vi "TeachHSLColor.vi"(7 "error in (no error)":errorcluster, 9 "ROI Descriptor":T2 {"Contours"."Type" items=["No Selection", "Point", "Line", "Rectangle", "Oval", "Polygon", "Freehand Region", "Annulus", "Unused2", "Unused3", "Broken Line", "Freehand Line", "Rotated Rectangle"]}, 10 "Image in":T1) -> (0 "error out":errorcluster, 1 "SatLimits":cluster{"Lower value":u8, "Upper value":u8}, 3 "HueLimits":cluster{"Lower value":u8, "Upper value":u8})   [LabVIEW 2015]
uses:
  <vilib>/vision/Image Controls.llb/IMAQ Image.ctl
  <vilib>/vision/NI_Vision_Development_Module.lvlib
panel:
  out "Sat":u32[](graph)
  out "Hue":u32[](graph)
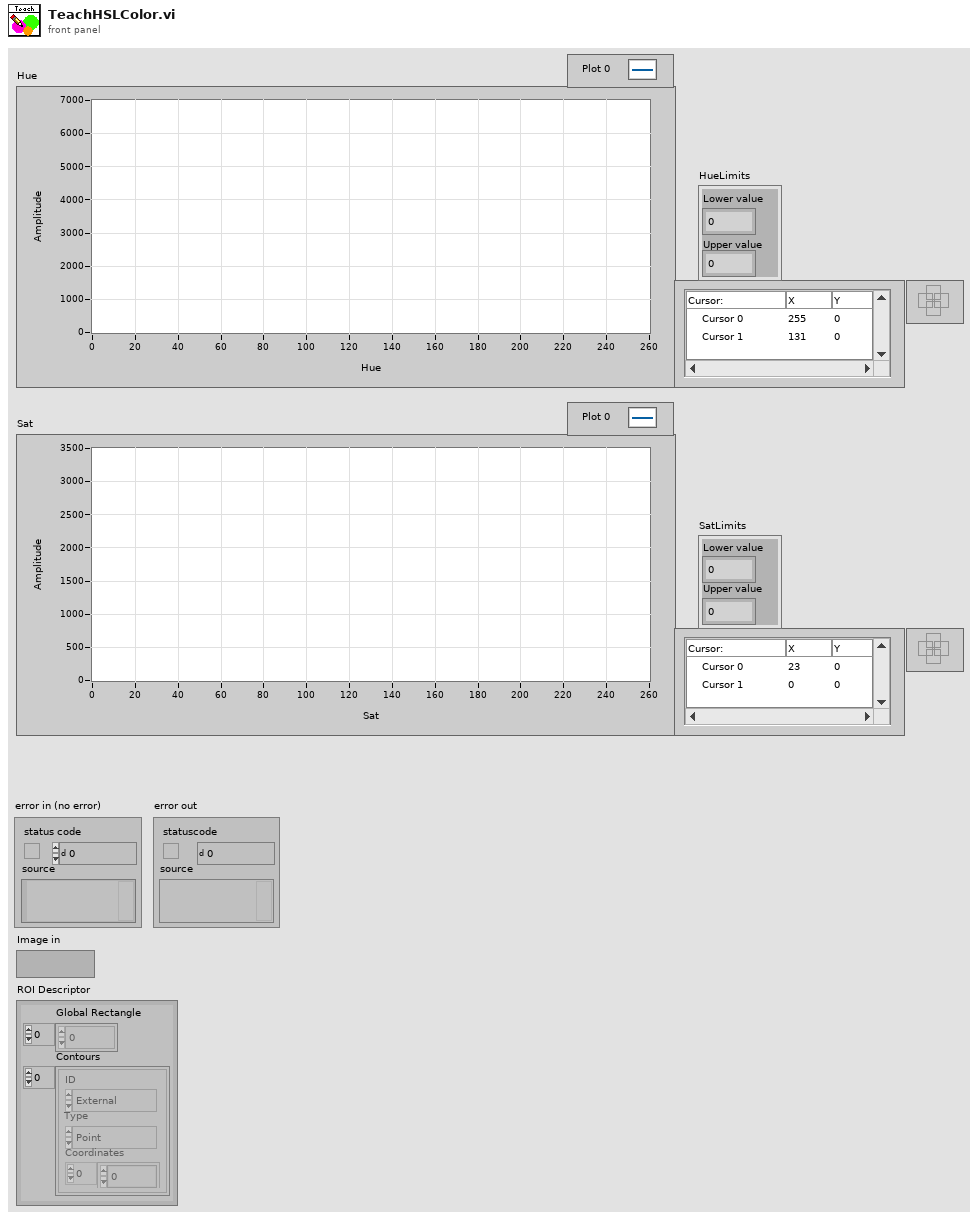
[diagram p1: front panel]
types:
  T1 = typedef "IMAQ Image.ctl" = refnum<image>
  T2 = typedef "ROI Descriptor" = cluster{"Global Rectangle":i32[], "Contours":cluster{"ID":enum32{"External", "Internal"}, "Type":u32, "Coordinates":i32[]}[]}
  T3 = typedef "Image Type" = u32
  T4 = cluster{"histogram":u32[], "Minimal Value":sgl, "Maximal Value":sgl, "Starting Value":sgl, "Interval Width":sgl, "Mean Value":sgl, "Standard  Variation":sgl, "Area (pixels)":i32}
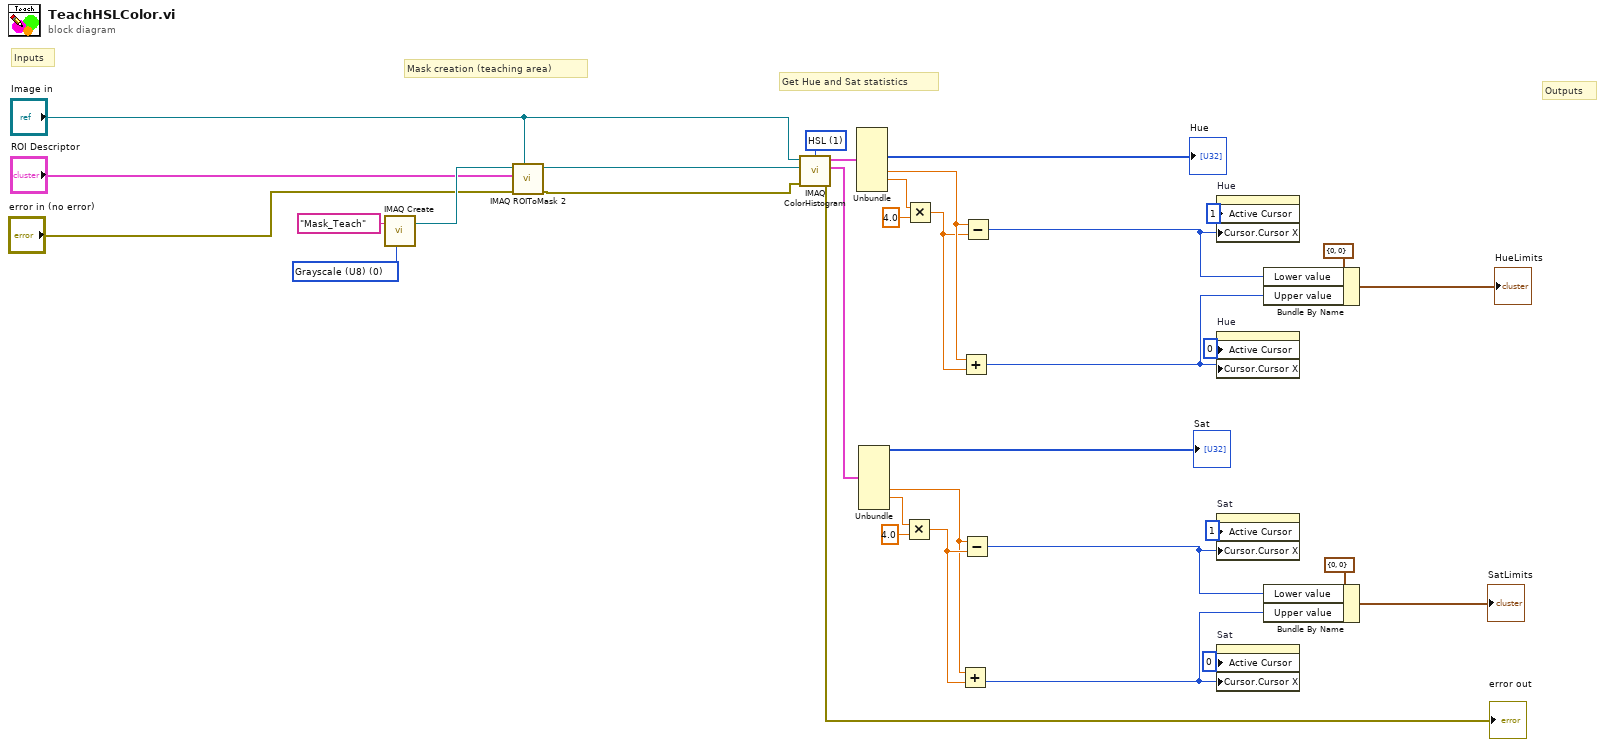
[diagram p0: block diagram]
diagram:
  w29 = u16 1 items=["RGB", "HSL", "HSV", "HSI", "CIE L*a*b*", "CIE XYZ"] ("Color Mode")
  w31 = T3 0 items=["Grayscale (U8)", "Grayscale (I16)", "Grayscale (SGL)", "Complex (CSG)", "RGB (U32)", "HSL (U32)", "RGB (U64)", "Grayscale (U16)"] ("Image Type")
  # "Outputs"
  # "Get Hue and Sat statistics"
  # "Mask creation (teaching area)"
  # "Inputs"
  n1 = call "IMAQ Create"("Image Name"="Mask_Teach", "Image Type"=w31) -> ("New Image"=w32:T1)  [unwired: 3 in, 1 out]
  n2 = call "IMAQ ROIToMask 2"("Image Model"="Image in", "error in (no error)"="error in (no error)", "ROI Descriptor"="ROI Descriptor", "Image"=w32) -> ("error out"=w33:errorcluster, "Image Out"=w34:T1)  [unwired: 5 in, 1 out]
  n3 = call "IMAQ ColorHistogram"("Color Mode"=w29, "Image Src"="Image in", "Image Mask"=w34, "error in (no error)"=w33) -> ("Red or Hue or X or L* Histogram Report"=w28:T4, "Green or Sat or Y or a* Histogram Report"=w25:T4, "error out"=→"error out":errorcluster)  [unwired: 2 in, 1 out]
  n4 = Unbundle(w28) -> ("histogram"=→"Hue":u32[], "Mean Value"=w15:sgl, "Standard  Variation"=w22:sgl)  [unwired: 5 out]
  n5 = Unbundle(w25) -> ("histogram"=→"Sat":u32[], "Mean Value"=w3:sgl, "Standard  Variation"=w2:sgl)  [unwired: 5 out]
  n6 = Multiply(x=w2, y=sgl 4.0) -> (x*y=w9:sgl)
  n7 = Multiply(x=w22, y=sgl 4.0) -> (x*y=w14:sgl)
  n8 = Add ("Addieren")(x=w3, y=w9) -> (x+y=w6:u8)
  n9 = Add ("Addieren")(x=w15, y=w14) -> (x+y=w12:u8)
  n10 = Subtract ("Subtrahieren")(x=w3, y=w9) -> (x-y=w7:u8)
  n11 = Subtract ("Subtrahieren")(x=w15, y=w14) -> (x-y=w13:u8)
  n12 = property on="Hue" class="WFGraph (strict)"("Active Cursor"=u32 1 ("Aktiver Cursor"), "Cursor.Cursor X"=w13) -> ()  [unwired: 2 in, 2 out]
  n13 = property on="Hue" class="WFGraph (strict)"("Active Cursor"=u32 0 ("Aktiver Cursor"), "Cursor.Cursor X"=w12) -> ()  [unwired: 2 in, 2 out]
  n14 = property on="Sat" class="WFGraph (strict)"("Active Cursor"=u32 1 ("Aktiver Cursor"), "Cursor.Cursor X"=w7) -> ()  [unwired: 2 in, 2 out]
  n15 = property on="Sat" class="WFGraph (strict)"("Active Cursor"=u32 0 ("Aktiver Cursor"), "Cursor.Cursor X"=w6) -> ()  [unwired: 2 in, 2 out]
  n16 = Bundle By Name(cluster=cluster{"Lower value":u8, "Upper value":u8} {"Lower value"=0, "Upper value"=0}, "Lower value"=w13, "Upper value"=w12) -> (→"HueLimits":cluster{"Lower value":u8, "Upper value":u8})
  n17 = Bundle By Name(cluster=cluster{"Lower value":u8, "Upper value":u8} {"Lower value"=0, "Upper value"=0}, "Lower value"=w7, "Upper value"=w6) -> (→"SatLimits":cluster{"Lower value":u8, "Upper value":u8})
